vi "test_Util_Transform.vi"(8 "error in (no error)":errorcluster) -> (0 "error out":errorcluster, 3 "Test Passed":bool)   [LabVIEW 2019]
uses:
  <vilib>/Rock Robotics/WPI/ThirdParty/JAS_Junk/TrajLib/TypeDef/POSE2D.ctl
  <vilib>/Rock Robotics/WPI/ThirdParty/JAS_Junk/TrajLib/TypeDef/TRANSLATION2D.ctl
  <vilib>/Rock Robotics/WPI/ThirdParty/JAS_Junk/TrajLib/TypeDef/ROTATION2D.ctl
  <vilib>/Rock Robotics/WPI/ThirdParty/JAS_Junk/TrajLib/Rotation2d_CreateAngle.vi
  <vilib>/Rock Robotics/WPI/ThirdParty/PhotonVisionLib/PhotonVisionLib.lvlib
  <vilib>/Rock Robotics/WPI/ThirdParty/JAS_Junk/TrajLib/Trajectory_Library.lvlib
panel:
  out "Test 1 Passed":bool
  out "Test 0 Passed":bool
  out "EstimateFieldToRobot 2":T1={"TRANSLATION"={"X"=0.0, "Y"=0.0}, "ROTATION"={"VALUE"=0.0, "COS"=1.0, "SIN"=0.0}} {"ROTATION"."SIN" format="%13.4f"; "ROTATION"."COS" format="%13.4f"; "ROTATION"."VALUE" format="%13.4f"; "TRANSLATION"."Y" format="%14.3f"; "TRANSLATION"."X" format="%14.3f"}
  out "EstimateFieldToRobot":T1={"TRANSLATION"={"X"=0.0, "Y"=0.0}, "ROTATION"={"VALUE"=0.0, "COS"=1.0, "SIN"=0.0}} {"ROTATION"."SIN" format="%13.4f"; "ROTATION"."COS" format="%13.4f"; "ROTATION"."VALUE" format="%13.4f"; "TRANSLATION"."Y" format="%14.3f"; "TRANSLATION"."X" format="%14.3f"}
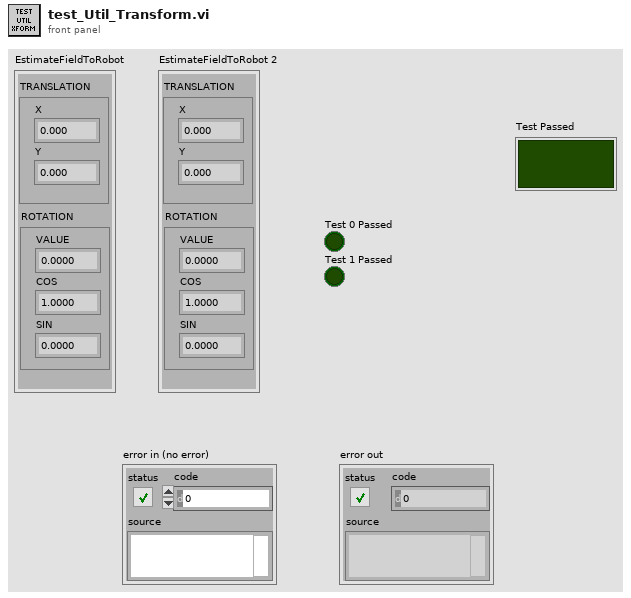
[diagram p1: front panel]
types:
  T1 = typedef "Trajectory_Library.lvlib/POSE2D.ctl" = cluster{"TRANSLATION":T2, "ROTATION":T3}
  T2 = typedef "Trajectory_Library.lvlib/TRANSLATION2D.ctl" = cluster{"X":dbl, "Y":dbl}
  T3 = typedef "Trajectory_Library.lvlib/ROTATION2D.ctl" = cluster{"VALUE":dbl, "COS":dbl, "SIN":dbl}
  T4 = typedef "Trajectory_Library.lvlib/TRANSFORM2D.ctl" = cluster{"TRANSLATION":T2, "ROTATION":T3, "xF":bool}
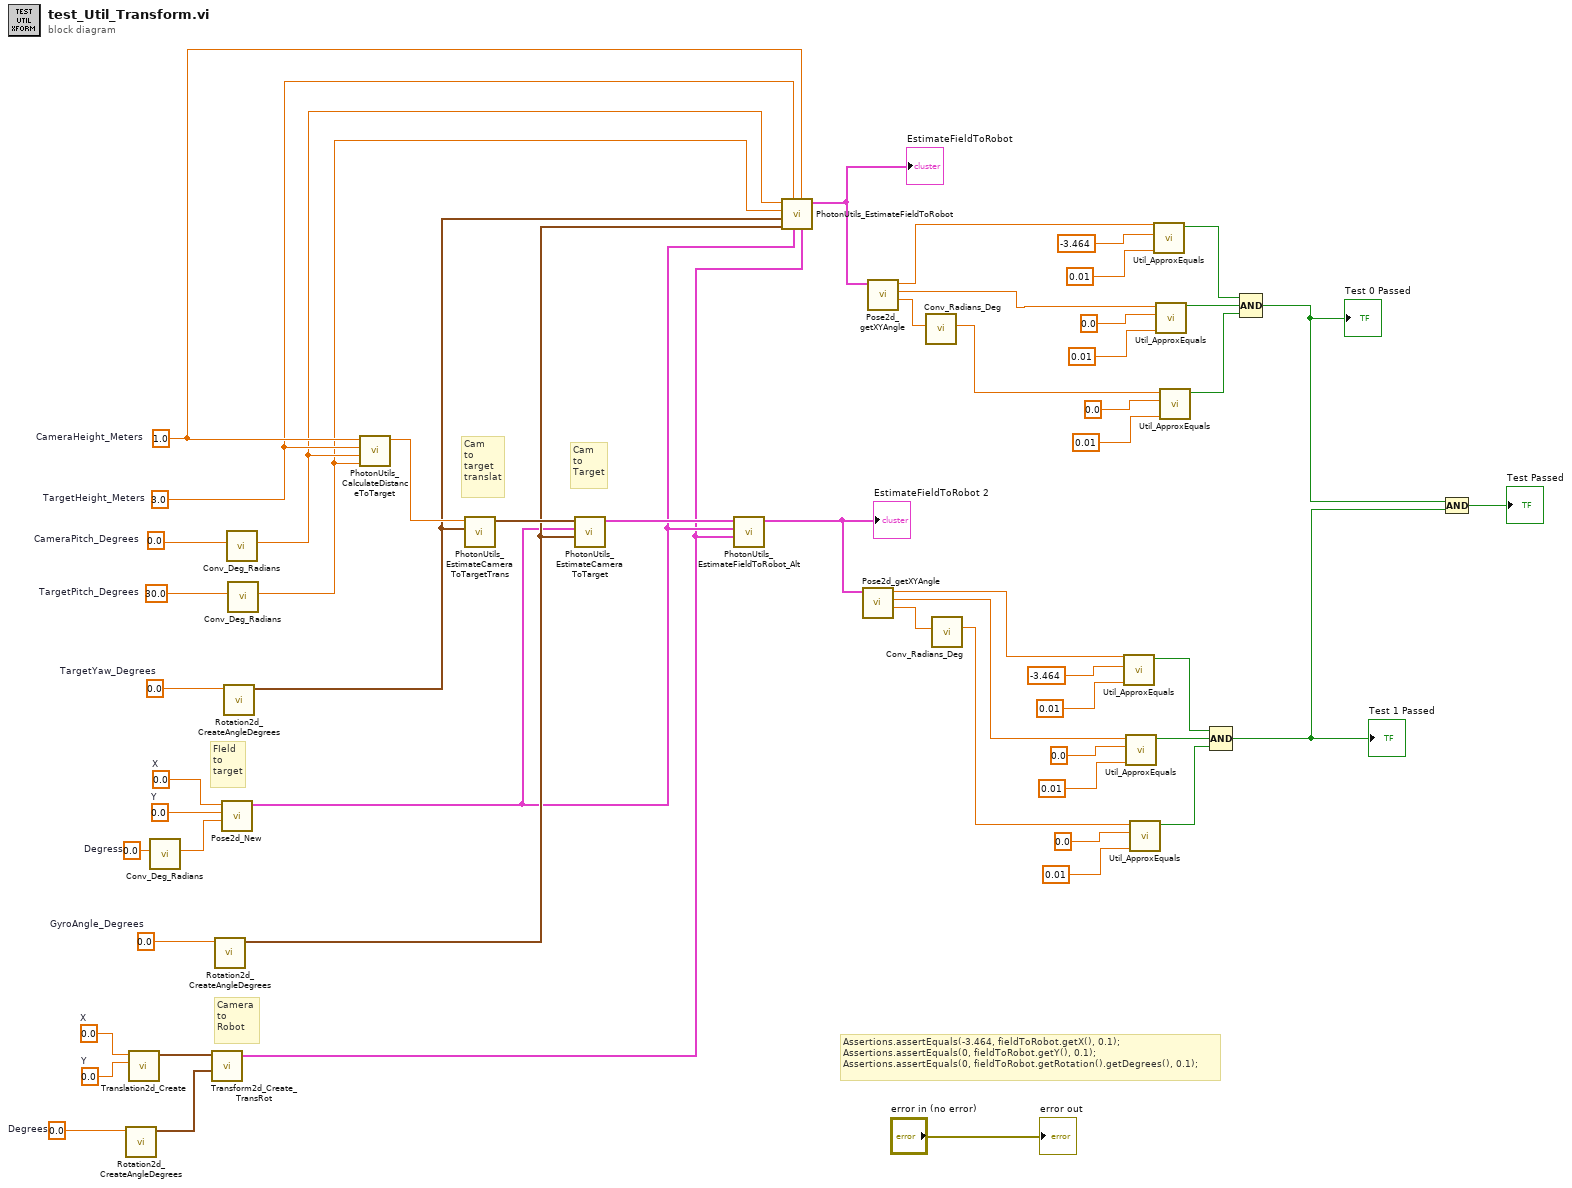
[diagram p0: block diagram]
diagram:
  w40 = 0.0  # X
  w41 = 0.0  # Y
  w43 = 0.0  # Degrees
  w46 = 0.0  # GyroAngle_Degrees
  w47 = 0.0  # Degress
  w49 = 0.0  # X
  w50 = 0.0  # Y
  w52 = 0.0  # TargetYaw_Degrees
  w35 = 1.0  # CameraHeight_Meters
  w34 = 3.0  # TargetHeight_Meters
  w55 = 0.0  # CameraPitch_Degrees
  w54 = 30.0  # TargetPitch_Degrees
  # "Assertions.assertEquals(-3.464, fieldToRobot.getX(), 0.1);\nAssertions.assertEquals(0, fieldToRobot.getY(), 0.1);\nAssertions.assertEquals(0, fieldToRobot.getRotation().getDegrees(), 0.1);"
  # "Camera\nto\nRobot"
  # "Cam\nto\nTarget"
  # "FIeld\nto\ntarget"
  # "Cam\nto\ntarget\ntranslat"
  n1 = call <vilib>:"Rotation2d_CreateAngleDegrees.vi"("Angle_Degrees"=w43) -> ("ROTATION"=w42:T3)  [unwired: 10 in]
  n2 = call <vilib>:"Translation2d_Create.vi"("Y"=w41, "X"=w40) -> ("TRANSLATION"=w44:T2)  [unwired: 9 in]
  n3 = call <vilib>:"Conv_Deg_Radians.vi"("Degress"=w47) -> ("Radians"=w48:dbl)  [unwired: 10 in]
  n4 = call <vilib>:"Transform2d_Create_TransRot.vi"("ROTATION"=w42, "TRANSLATION"=w44) -> ("TRANSFORM"=w36:T4)  [unwired: 9 in]
  n5 = call <vilib>:"Rotation2d_CreateAngleDegrees.vi"("Angle_Degrees"=w46) -> ("ROTATION"=w38:T3)  [unwired: 10 in]
  n6 = call <vilib>:"Pose2d_New.vi"("Heading"=w48, "Y"=w50, "X"=w49) -> ("out POSe"=w37:T1)  [unwired: 8 in]
  n7 = call <vilib>:"Rotation2d_CreateAngleDegrees.vi"("Angle_Degrees"=w52) -> ("ROTATION"=w39:T3)  [unwired: 10 in]
  n8 = call <vilib>:"Conv_Deg_Radians.vi"("Degress"=w55) -> ("Radians"=w33:dbl)  [unwired: 10 in]
  n9 = call <vilib>:"Conv_Deg_Radians.vi"("Degress"=w54) -> ("Radians"=w32:dbl)  [unwired: 10 in]
  n10 = call <vilib>:"PhotonUtils_CalculateDistanceToTarget.vi"("TargetPitch_Radians"=w32, "CameraPitch_Radians"=w33, "TargetHeight_Meters"=w34, "CameraHeight_Meters"=w35) -> ("DistanceToTarget_Meters"=w53:dbl)  [unwired: 7 in]
  n11 = call <vilib>:"PhotonUtils_EstimateCameraToTargetTrans.vi"("Yaw"=w39, "TargetDistance_Meters"=w53) -> ("CameraToTarget"=w51:T2)  [unwired: 9 in]
  n12 = call <vilib>:"PhotonUtils_EstimateCameraToTarget.vi"("GyroAngle"=w38, "FieldToTarget"=w37, "CameraToTargetTranslation"=w51) -> ("estimateCameraToTarget"=w45:T4)  [unwired: 8 in]
  n13 = call <vilib>:"PhotonUtils_EstimateFieldToRobot_Alt.vi"("CameraToRobot"=w36, "FieldToTarget"=w37, "CameraToTarget,"=w45) -> ("EstimateFieldToRobot"=w31:T1)  [unwired: 8 in]
  "EstimateFieldToRobot 2" <- w31
  n14 = call <vilib>:"PhotonUtils_EstimateFieldToRobot.vi"("CameraToRobot"=w36, "cameraHeight_Meters"=w35, "FieldToTarget"=w37, "targetHeight_Meters"=w34, "GyroAngle"=w38, "TargetYaw"=w39, "targetPitch_Radians"=w32, "cameraPitch_Radians"=w33) -> ("EstimateFieldToRobot"=w30:T1)  [unwired: 3 in]
  "EstimateFieldToRobot" <- w30
  n15 = call <vilib>:"Pose2d_getXYAngle.vi"("in POSE"=w31) -> ("Angle"=w23:dbl, "Y"=w21:dbl, "X"=w22:dbl)  [unwired: 8 in]
  n16 = call <vilib>:"Pose2d_getXYAngle.vi"("in POSE"=w30) -> ("Angle"=w13:dbl, "Y"=w10:dbl, "X"=w11:dbl)  [unwired: 8 in]
  n17 = call <vilib>:"Conv_Radians_Deg.vi"("Radians"=w13) -> ("Degrees"=w12:dbl)  [unwired: 10 in]
  n18 = call <vilib>:"Conv_Radians_Deg.vi"("Radians"=w23) -> ("Degrees"=w20:dbl)  [unwired: 10 in]
  n19 = call <vilib>:"Util_ApproxEquals.vi"("Tolerance"=0.01, "Value 2"=-3.464, "Value 1"=w22) -> ("ApproxEquals"=w6:bool)  [unwired: 8 in]
  n20 = call <vilib>:"Util_ApproxEquals.vi"("Tolerance"=0.01, "Value 2"=0.0, "Value 1"=w21) -> ("ApproxEquals"=w5:bool)  [unwired: 8 in]
  n21 = call <vilib>:"Util_ApproxEquals.vi"("Tolerance"=0.01, "Value 2"=0.0, "Value 1"=w20) -> ("ApproxEquals"=w4:bool)  [unwired: 8 in]
  n22 = call <vilib>:"Util_ApproxEquals.vi"("Tolerance"=0.01, "Value 2"=-3.464, "Value 1"=w11) -> ("ApproxEquals"=w9:bool)  [unwired: 8 in]
  n23 = call <vilib>:"Util_ApproxEquals.vi"("Tolerance"=0.01, "Value 2"=0.0, "Value 1"=w10) -> ("ApproxEquals"=w8:bool)  [unwired: 8 in]
  n24 = call <vilib>:"Util_ApproxEquals.vi"("Tolerance"=0.01, "Value 2"=0.0, "Value 1"=w12) -> ("ApproxEquals"=w7:bool)  [unwired: 8 in]
  n25 = Compound Arithmetic op=AND(w6, w5, w4) -> (w1:bool)
  "Test 1 Passed" <- w1
  n26 = Compound Arithmetic op=AND(w9, w8, w7) -> (w2:bool)
  "Test 0 Passed" <- w2
  n27 = Compound Arithmetic op=AND(w2, w1) -> (→"Test Passed":bool)
  "error out" <- "error in (no error)"
